vi "Configure Analog Output Mode.vi"(8 "error in (no error)":errorcluster, 10 "Analog Output Mode (0: Disabled)":i32(ring) items=["Disabled", "Parallel", "Series"], 11 "VISA resource name":refnum<visa-resource-name>) -> (0 "error out":errorcluster, 3 "VISA resource name out":refnum<visa-resource-name>)   [LabVIEW 2018, in "XP Power PLS600.lvlib"]
doc: "Sets the analog output mode for the ENET-IFC board."
uses:
  XP Power PLS600.lvlib
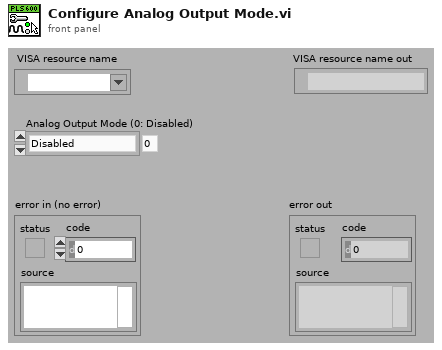
[diagram p1: front panel]
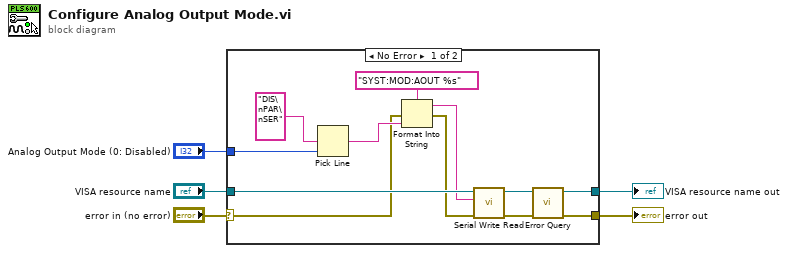
[diagram p0: block diagram]
diagram:
  n1 = case shown="No Error" "error in (no error)" {
    selector: "error in (no error)" -> [w8 w18]
    tunnel: "Analog Output Mode (0: Disabled)" -> [w16 _]
    tunnel: [w15 w19] -> w4
    tunnel: [w14 w18] -> w3
    tunnel: "VISA resource name" -> [w13 w19]
    frame No Error {
      n2 = Pick Line(multi-line string="DIS\nPAR\nSER", line index=w16) -> (output string=w9:string)  [unwired: 1 in]
      n3 = Format Into String(format string="SYST:MOD:AOUT %s" ("Command to Send"), error in=w8, w9) -> (resulting string=w6:string, error out=w7:errorcluster)  [unwired: 1 in]
      n4 = call "Serial Write Read.vi"("error in (no error)"=w7, "Write Buffer"=w6, "VISA resource name"=w13) -> ("error out"=w11:errorcluster, "VISA resource name out"=w12:refnum<visa-resource-name>)  [unwired: 6 in, 1 out]
      n5 = call "Error Query.vi"("error in (no error)"=w11, "VISA resource name"=w12) -> ("error out"=w14:errorcluster, "VISA resource name out"=w15:refnum<visa-resource-name>)  [unwired: 6 in, 2 out]
    }
    frame Error {
    }
  }
  "VISA resource name out" <- w4
  "error out" <- w3
